vi "One note refresh.vi"(8 "error in (no error)":errorcluster, 9 "Refresh Token In":string, 11 "Authorization Code In":string) -> (0 "error out":errorcluster, 1 "Refresh Token Out":string, 2 "Access Token Out":string, 3 "Authorization Code Out":string)   [LabVIEW 2016]
uses:
  <vilib>/httpClient/POSTBuffer.vi
  <vilib>/httpClient/LabVIEWHTTPClient.lvlib
  <vilib>/LVH/i3 JSON/i3-json.lvlib
  <vilib>/LVH/i3 JSON/JSON Parsing/Get Object Parameter Files/Get Object Parameter - String.vi
  <vilib>/addons/_JKI.lib/Serialization/JSON/JKI JSON Serialization.lvlib
  REST_APIs/src/Joe/Object Oriented Version/Response/Response.lvclass
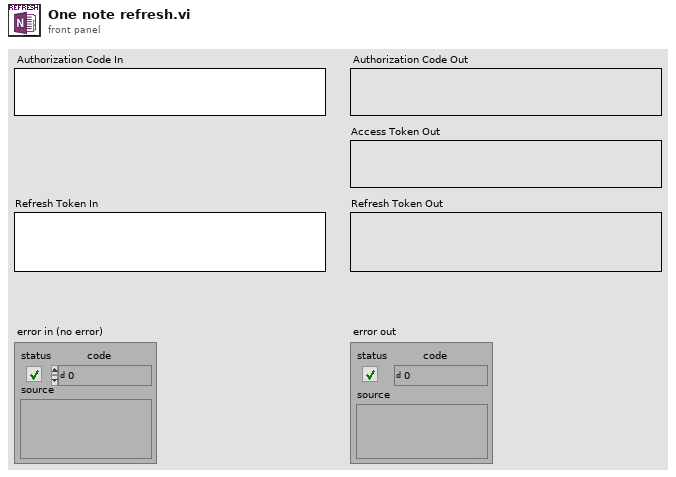
[diagram p1: front panel]
types:
  T1 = typedef "LabVIEWHTTPClient.lvlib/ClientHandle.ctl" = refnum<k1>
  T2 = cluster{"token_type":string, "scope":string, "access_token":string, "refresh_token":string, "user_id":string, "expires_in":i32}
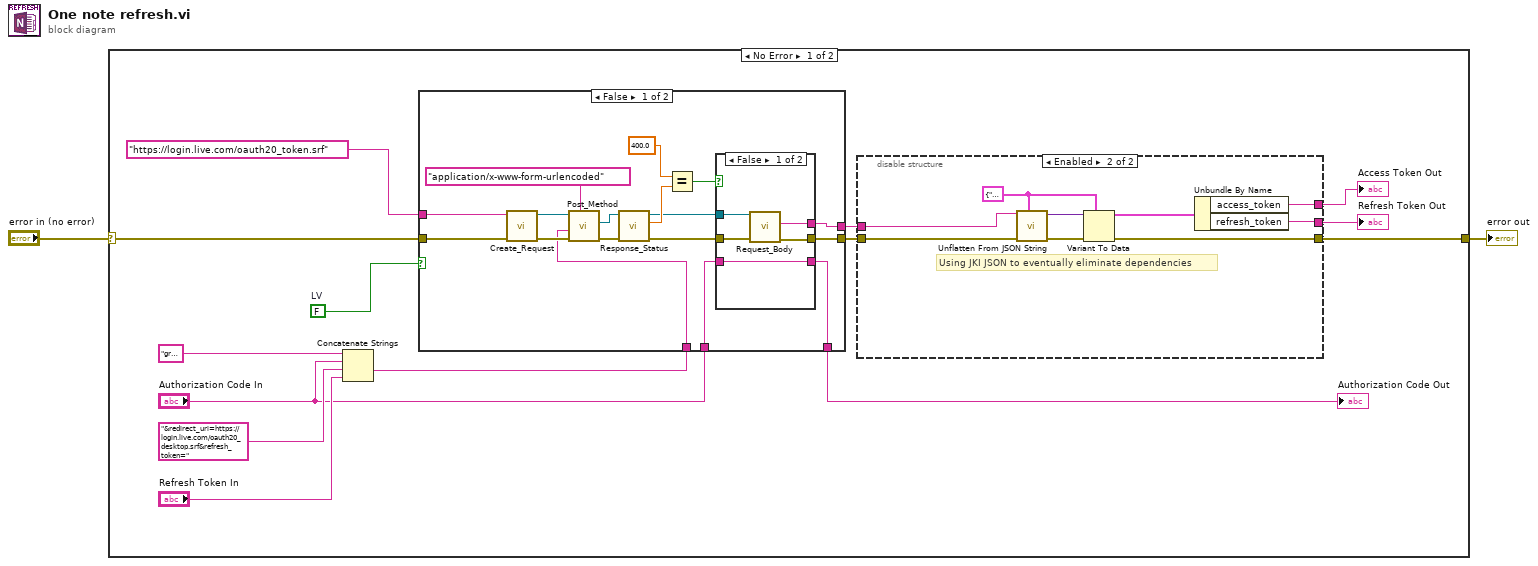
[diagram p0: block diagram]
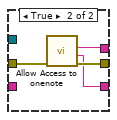
[diagram p2: hidden frame]
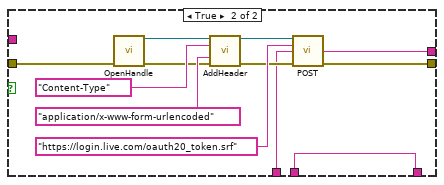
[diagram p3: hidden frame]
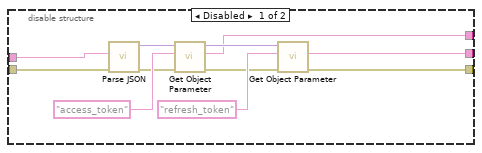
[diagram p4: hidden frame]
diagram:
  n1 = case shown="No Error" "error in (no error)" {
    selector: "error in (no error)" -> [w8 w75]
    tunnel: [w9 w75] -> w1
    frame No Error {
      w4 = FALSE  # LV
      n2 = Concatenate Strings("grant_type=refresh_token&client_id=c698ce01-75b1-4eb8-b040-9787b75e6b48&code=" ("string"), "Authorization Code In", "&redirect_uri=https://login.live.com/oauth20_desktop.srf&refresh_token=", "Refresh Token In") -> (w3:string)
      n3 = case shown="False" w4 {
        tunnel: [w22 w49] -> w13
        tunnel: [w24 w46] -> w12
        tunnel: w8 -> [w31 w45]
        tunnel: "https://login.live.com/oauth20_token.srf" ("url") -> [w32 _]
        tunnel: "Authorization Code In" -> [w20 w43]
        tunnel: [w19 w43] -> w5
        tunnel: w3 -> [w18 w44]
        frame False {
          n4 = call "Create_Request.vi"("error in (no error)"=w31, "Base URL"=w32) -> ("error out"=w30:errorcluster, "Request out"=w33:refnum<class "Request.lvclass">)  [unwired: 8 in]
          n5 = call "Post_Method.vi"("Body Content-Type"="application/x-www-form-urlencoded", "error in (no error)"=w30, "Body"=w18, "Request in"=w33) -> ("error out"=w29:errorcluster, "Response out"=w28:refnum<class "Response.lvclass">)  [unwired: 5 in, 1 out]
          n6 = call "Response_Status.vi"("error in (no error)"=w29, "Response in"=w28) -> ("error out"=w25:errorcluster, "Status Code"=w27:dbl, "Response out"=w21:refnum<class "Response.lvclass">)  [unwired: 6 in, 1 out]
          n7 = Equal?(x=400.0, y=w27) -> (x = y?=w23:bool)
          n8 = case shown="False" w23 {
            tunnel: [w37 w41] -> w24
            tunnel: w25 -> [w38 w42]
            tunnel: [w35 w40] -> w22
            tunnel: w21 -> [w36 _]
            tunnel: w20 -> [w34 _]
            tunnel: [w34 w39] -> w19
            frame False {
              n9 = call "Request_Body.vi"("error in (no error)"=w38, "Response in"=w36) -> ("error out"=w37:errorcluster, "Response Body"=w35:string)  [unwired: 7 in, 1 out]
            }
            frame True {
              n10 = call "Allow Access to onenote.vi"("error in (no error)"=w42) -> ("error out"=w41:errorcluster, "Authorization Code"=w39:string, "body"=w40:string)  [unwired: 8 in]
            }
          }
        }
        frame True {
          n11 = call <vilib>:"OpenHandle.vi"("error in (no error)"=w45) -> ("client handle out"=w54:T1, "error out"=w48:errorcluster)  [unwired: 13 in]
          n12 = call <vilib>:"AddHeader.vi"("client handle"=w54, "header"="Content-Type", "value"="application/x-www-form-urlencoded", "error in (no error)"=w48) -> ("client handle out"=w50:T1, "error out"=w47:errorcluster)  [unwired: 10 in]
          n13 = call-poly <vilib>:"POST.vi"("client handle"=w50, "url"="https://login.live.com/oauth20_token.srf", "buffer"=w44, "error in (no error)"=w47) -> ("body"=w49:string, "error out"=w46:errorcluster)  [unwired: 8 in, 2 out]
        }
      }
      "Authorization Code Out" <- w5
      n14 = disable-structure shown="Enabled" {
        disable-tunnel: w13 -> [w61 w70]
        disable-tunnel: w12 -> [w60 w71]
        disable-tunnel: [w57 w68] -> w11
        disable-tunnel: [w56 w67] -> w10
        disable-tunnel: [w55 w66] -> w9
        frame Disabled {
          n15 = call <vilib>:"Parse JSON.vi"("error in (no error)"=w60, "JSON String"=w61) -> ("error out"=w59:errorcluster, "JSON Tree"=w64:variant)  [unwired: 6 in, 2 out]
          n16 = call-poly <vilib>:"Get Object Parameter.vi"("error in (no error)"=w59, "Parameter Name"="access_token", "JSON Tree In (JSON Object)"=w64) -> ("error out"=w58:errorcluster, "String Value"=w57:string, "JSON Tree Out Passthrough"=w63:variant)  [unwired: 5 in, 1 out]
          n17 = call-poly <vilib>:"Get Object Parameter.vi"("error in (no error)"=w58, "Parameter Name"="refresh_token", "JSON Tree In (JSON Object)"=w63) -> ("error out"=w55:errorcluster, "String Value"=w56:string)  [unwired: 5 in, 2 out]
        }
        frame Enabled {
          w73 = T2 {"token_type"="", "scope"="", "access_token"="", "refresh_token"="", "user_id"="", "expires_in"=0}
          # "Using JKI JSON to eventually eliminate dependencies"
          n18 = call <vilib>:"Unflatten From JSON String.vi"("Type and Defaults"=w73, "error in (no error)"=w71, "JSON String"=w70) -> ("error out"=w74:errorcluster, "Variant"=w72:variant)  [unwired: 7 in]
          n19 = Variant To Data(error in=w74, type=w73, Variant=w72) -> (data=w69:T2, error out=w66:errorcluster)
          n20 = Unbundle By Name(w69) -> ("access_token"=w68:string, "refresh_token"=w67:string)
        }
      }
      "Refresh Token Out" <- w10
      "Access Token Out" <- w11
    }
    frame Error {
    }
  }
  "error out" <- w1
